vi "sendMessage.vi"(8 "error in":errorcluster, 9 "data":variant, 10 "message":string, 11 "TaskController in":refnum<class "TaskController.lvclass">) -> (0 "error out":errorcluster, 3 "TaskController out":refnum<class "TaskController.lvclass">)   [LabVIEW 2023, in "TLC_Daemon.lvlib" / "TaskController.lvclass"]
uses:
  TaskController.lvclass
  TaskController.lvclass/TaskController.ctl
  ITaskChannel/ITaskChannel.lvclass
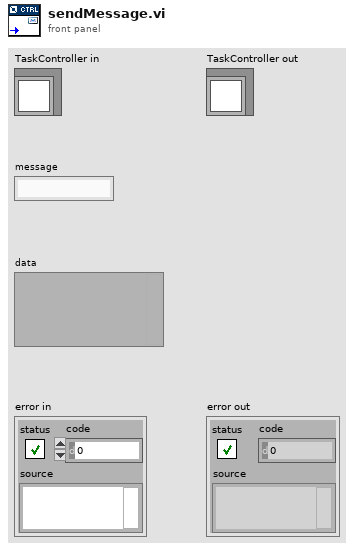
[diagram p1: front panel]
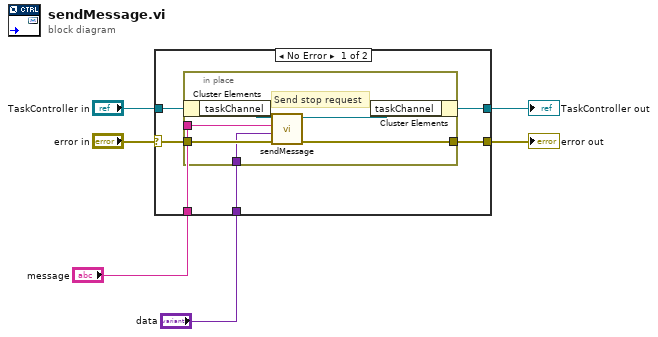
[diagram p0: block diagram]
diagram:
  n1 = case shown="No Error" "error in" {
    selector: "error in" -> [w9 w20]
    tunnel: [w11 w20] -> w3
    tunnel: [w12 w19] -> w4
    tunnel: "TaskController in" -> [w10 w19]
    tunnel: "message" -> [w8 _]
    tunnel: "data" -> [w7 _]
    frame No Error {
      n2 = in-place {
        in-place-border: w9 -> [w18]
        in-place-border: [w17] -> w11
        in-place-border: w8 -> [w14]
        in-place-border: w7 -> [w13]
        # "Send stop request"
        n3 = in-place-cluster #1(w10) -> ("taskChannel"=w16:refnum<class "ITaskChannel.lvclass">)
        n4 = call-dynamic "sendMessage.vi"("error in (no error)"=w18, "data"=w13, "message"=w14, "ITaskChannel in"=w16) -> ("error out"=w17:errorcluster, "ITaskChannel out"=w15:refnum<class "ITaskChannel.lvclass">)  [unwired: 6 in]
        n5 = in-place-cluster #1("taskChannel"=w15) -> (w12:refnum<class "TaskController.lvclass">)
      }
    }
    frame Error {
    }
  }
  "error out" <- w3
  "TaskController out" <- w4
